vi "Shift Register bkp2.vi"(6 "Rxy in":T1, 7 "load":bool, 8 "shift":bool) -> (5 "Rxy out":u64)   [LabVIEW 2017]
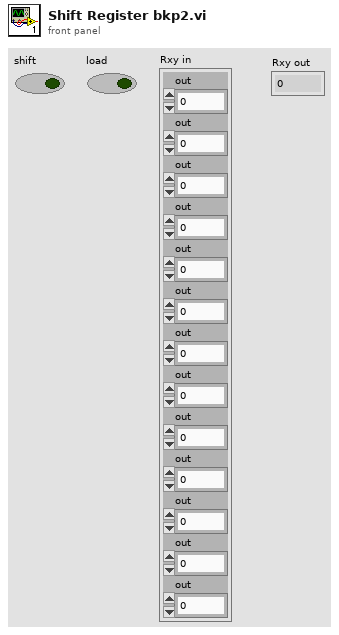
[diagram p1: front panel]
types:
  T1 = cluster{"out":u64, "out":u64, "out":u64, "out":u64, "out":u64, "out":u64, "out":u64, "out":u64, "out":u64, "out":u64, "out":u64, "out":u64, "out":u64}
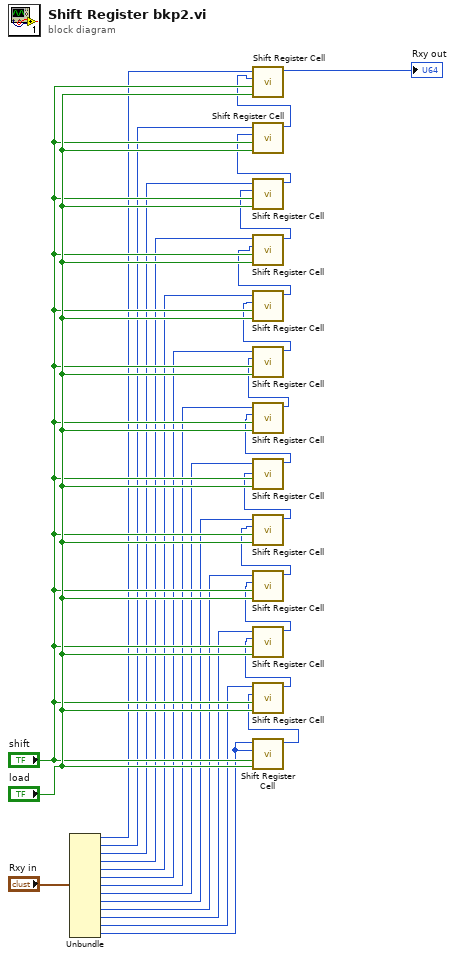
[diagram p0: block diagram]
diagram:
  n1 = Unbundle("Rxy in") -> ("out"=w15:u64, "out"=w16:u64, "out"=w17:u64, "out"=w18:u64, "out"=w19:u64, "out"=w20:u64, "out"=w21:u64, "out"=w22:u64, "out"=w23:u64, "out"=w24:u64, "out"=w25:u64, "out"=w26:u64, "out"=w1:u64)
  n2 = call "Shift Register Cell.vi"("load"="load", "shift"="shift", "Rxy shift"=w1, "Rxy load"=w1) -> ("Rxy"=w14:u64)  [unwired: 7 in]
  n3 = call "Shift Register Cell.vi"("load"="load", "shift"="shift", "Rxy shift"=w14, "Rxy load"=w26) -> ("Rxy"=w13:u64)  [unwired: 7 in]
  n4 = call "Shift Register Cell.vi"("load"="load", "shift"="shift", "Rxy shift"=w13, "Rxy load"=w25) -> ("Rxy"=w12:u64)  [unwired: 7 in]
  n5 = call "Shift Register Cell.vi"("load"="load", "shift"="shift", "Rxy shift"=w12, "Rxy load"=w24) -> ("Rxy"=w11:u64)  [unwired: 7 in]
  n6 = call "Shift Register Cell.vi"("load"="load", "shift"="shift", "Rxy shift"=w11, "Rxy load"=w23) -> ("Rxy"=w10:u64)  [unwired: 7 in]
  n7 = call "Shift Register Cell.vi"("load"="load", "shift"="shift", "Rxy shift"=w10, "Rxy load"=w22) -> ("Rxy"=w9:u64)  [unwired: 7 in]
  n8 = call "Shift Register Cell.vi"("load"="load", "shift"="shift", "Rxy shift"=w9, "Rxy load"=w21) -> ("Rxy"=w8:u64)  [unwired: 7 in]
  n9 = call "Shift Register Cell.vi"("load"="load", "shift"="shift", "Rxy shift"=w8, "Rxy load"=w20) -> ("Rxy"=w7:u64)  [unwired: 7 in]
  n10 = call "Shift Register Cell.vi"("load"="load", "shift"="shift", "Rxy shift"=w7, "Rxy load"=w19) -> ("Rxy"=w6:u64)  [unwired: 7 in]
  n11 = call "Shift Register Cell.vi"("load"="load", "shift"="shift", "Rxy shift"=w6, "Rxy load"=w18) -> ("Rxy"=w5:u64)  [unwired: 7 in]
  n12 = call "Shift Register Cell.vi"("load"="load", "shift"="shift", "Rxy shift"=w5, "Rxy load"=w17) -> ("Rxy"=w4:u64)  [unwired: 7 in]
  n13 = call "Shift Register Cell.vi"("load"="load", "shift"="shift", "Rxy shift"=w4, "Rxy load"=w16) -> ("Rxy"=w3:u64)  [unwired: 7 in]
  n14 = call "Shift Register Cell.vi"("load"="load", "shift"="shift", "Rxy shift"=w3, "Rxy load"=w15) -> ("Rxy"=→"Rxy out":u64)  [unwired: 7 in]
